vi "OSSP_Problem_Read.vi"(8 "error in (no error)":errorcluster, 11 "OSSP_Problem.lvclass In":refnum<class "OSSP_Problem.lvclass">) -> (0 "error out":errorcluster, 3 "OSSP_Problem.lvclass Out":refnum<class "OSSP_Problem.lvclass">)   [LabVIEW 2013, in "OSSP_Problem.lvclass"]
uses:
  OSSP_Problem.lvclass
  OSSP_Problem.lvclass/OSSP_Problem.ctl
panel:
  out "Array":u16[][](array[numeric])
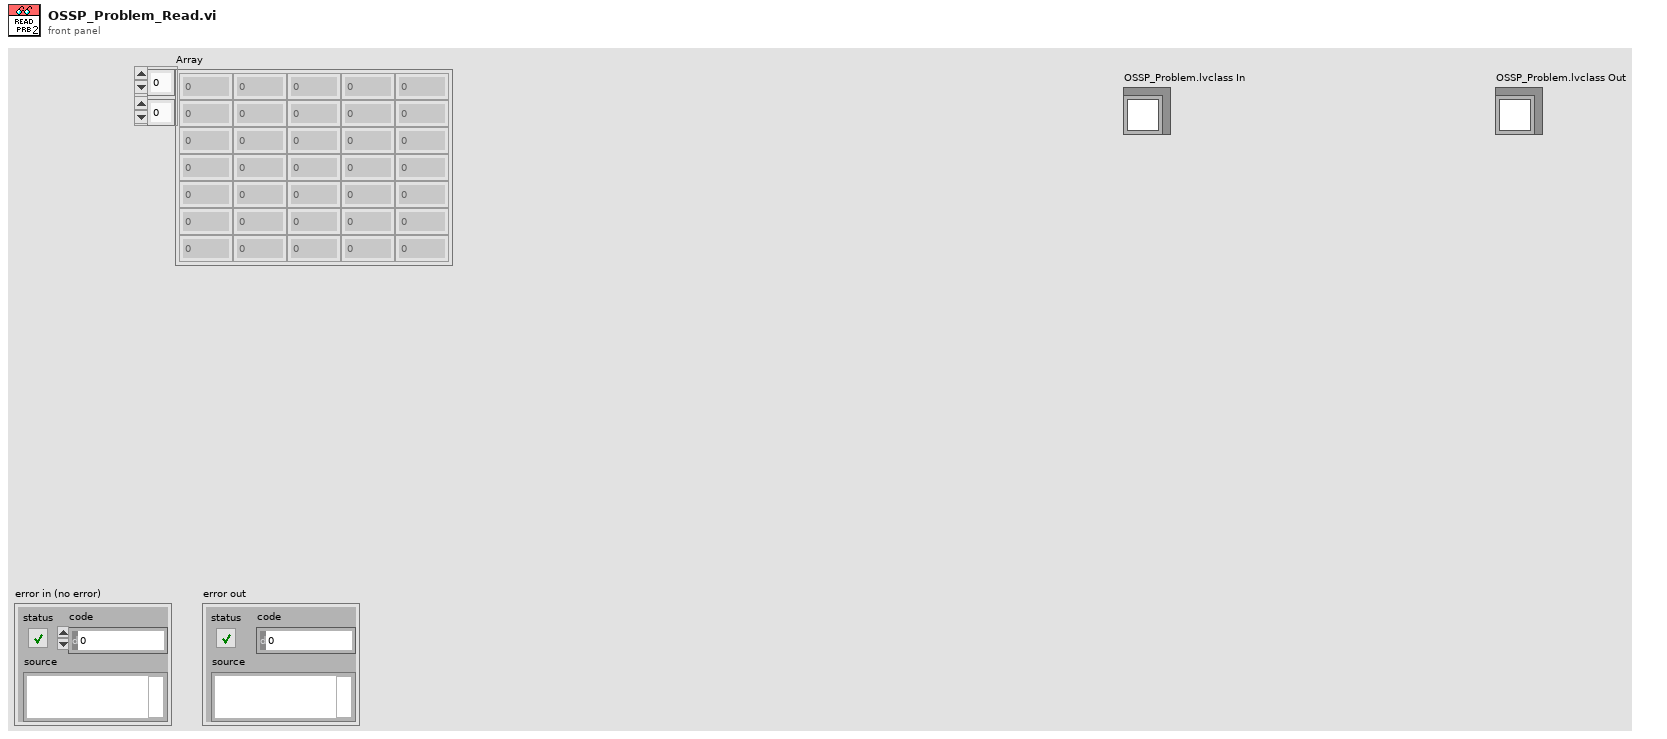
[diagram p1: front panel]
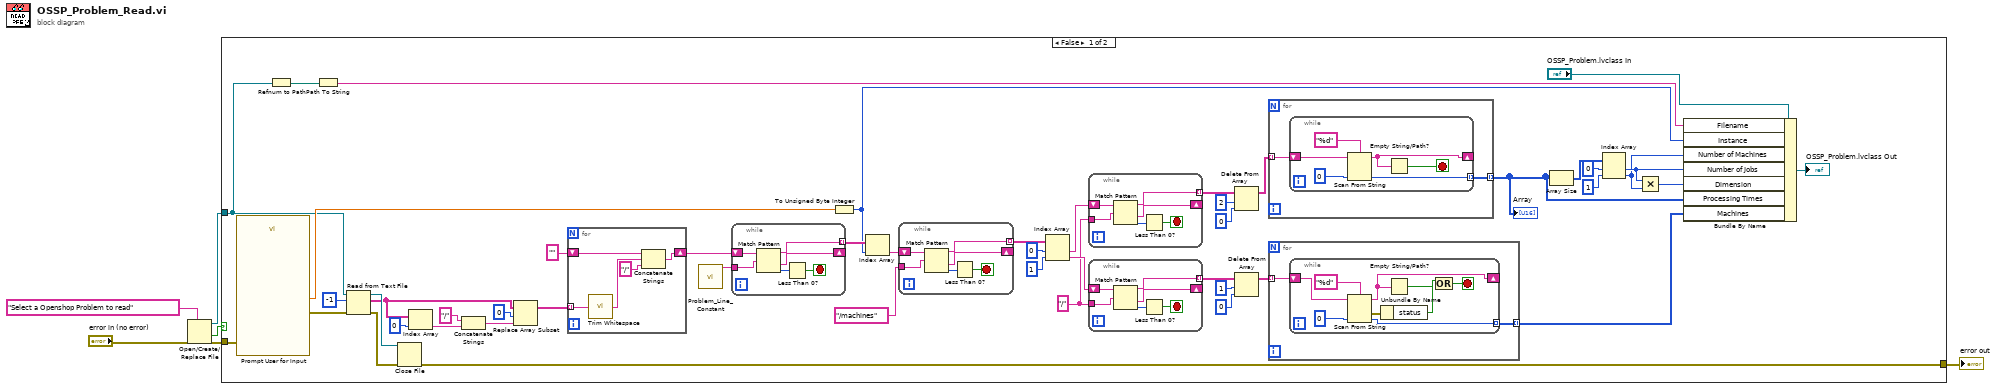
[diagram p0: block diagram]
diagram:
  n1 = Open/Create/Replace File(error in="error in (no error)", prompt="Select a Openshop Problem to read") -> (refnum out=w3:refnum<file>, cancelled=w2:bool, error out=w4:errorcluster)  [unwired: 4 in]
  n2 = case shown="False" w2 {
    tunnel: w4 -> [w51 w103]
    tunnel: w3 -> [w9 _]
    tunnel: [w10 w103] -> w1
    frame False {
      w27 = "/" ("Problem Line")
      n3 = call "Prompt User for Input"("error in (no error)"=w51) -> ("Instance Number"=w49:dbl, "error out"=w50:errorcluster)  [unwired: 16 in, 1 out]
      n4 = Refnum to Path(1:w9) -> (0:w8:path)
      n5 = Path To String(path=w8) -> (string=w7:string)
      n6 = Read from Text File(file (use dialog)=w9, count=-1, error in=w50) -> (refnum out=w53:refnum<file>, text=w44:string[], error out=w52:errorcluster)  [unwired: 1 in, 1 out]
      n7 = Close File(refnum=w53, error in=w52) -> (error out=w10:errorcluster)  [unwired: 1 out]
      n8 = Index Array(array=w44, index=0) -> (element=w47:string)
      n9 = Concatenate Strings("/" ("string"), w47) -> (w43:string)
      n10 = Replace Array Subset(array=w44, new element=w43, index=0) -> (w42:string[])
      n11 = for {
        tunnel: w42 -> [w94] mode=indexing
        shift-right: [w90] -> w40
        shift-left: "" -> [w93]
        n12 = call <vilib>:"Trim Whitespace.vi"("string"=w94) -> ("trimmed string"=w92:string)  [unwired: 1 in]
        n13 = Concatenate Strings(w93, w92, "/" ("string")) -> (w90:string)
      }
      n14 = call "Problem_Line_Constant.vi"() -> ("Problem Line"=w39:string)  [unwired: 11 in]
      n15 = while {
        tunnel: w39 -> [w88]
        shift-right: [w86] -> _
        shift-left: w40 -> [w89]
        tunnel: [w85] -> w38 mode=indexing
        stop <- w84 stop-if-true
        n16 = Match Pattern(string=w89, regular expression=w88) -> (before substring=w85:string, after substring=w86:string, offset past match=w87:i32)  [unwired: 1 in, 1 out]
        n17 = Less Than 0?(x=w87) -> (x < 0?=w84:bool)
      }
      n18 = To Unsigned Byte Integer(number=w49) -> (unsigned 8bit integer=w20:u8)
      n19 = Index Array(array=w38, index=w20) -> (element=w37:string)
      n20 = while {
        tunnel: "/machines" ("Problem Line") -> [w82]
        shift-right: [w80] -> _
        shift-left: w37 -> [w83]
        tunnel: [w79] -> w35 mode=indexing
        stop <- w78 stop-if-true
        n21 = Match Pattern(string=w83, regular expression=w82) -> (before substring=w79:string, after substring=w80:string, offset past match=w81:i32)  [unwired: 1 in, 1 out]
        n22 = Less Than 0?(x=w81) -> (x < 0?=w78:bool)
      }
      n23 = Index Array(array=w35, index #1=0 ("index"), index #2=1 ("index")) -> (element #1=w33:string, element #2=w28:string)
      n24 = while {
        tunnel: w27 -> [w76]
        shift-right: [w74] -> _
        shift-left: w33 -> [w77]
        tunnel: [w73] -> w32 mode=indexing
        stop <- w72 stop-if-true
        n25 = Match Pattern(string=w77, regular expression=w76) -> (before substring=w73:string, after substring=w74:string, offset past match=w75:i32)  [unwired: 1 in, 1 out]
        n26 = Less Than 0?(x=w75) -> (x < 0?=w72:bool)
      }
      n27 = while {
        tunnel: w27 -> [w70]
        shift-right: [w68] -> _
        shift-left: w28 -> [w71]
        tunnel: [w67] -> w26 mode=indexing
        stop <- w66 stop-if-true
        n28 = Match Pattern(string=w71, regular expression=w70) -> (before substring=w67:string, after substring=w68:string, offset past match=w69:i32)  [unwired: 1 in, 1 out]
        n29 = Less Than 0?(x=w69) -> (x < 0?=w66:bool)
      }
      n30 = Delete From Array(array=w32, length=2, index=0) -> (array with subset deleted=w23:string[])  [unwired: 1 out]
      n31 = Delete From Array(array=w26, length=1, index=0) -> (array with subset deleted=w22:string[])  [unwired: 1 out]
      n32 = for {
        tunnel: w23 -> [w96] mode=indexing
        tunnel: [w95] -> w12 mode=indexing
        n33 = while {
          shift-right: [w98] -> _
          shift-left: w96 -> [w102]
          tunnel: [w100] -> w95 mode=indexing
          stop <- w97 stop-if-true
          n34 = Scan From String(format string="%d", input string=w102, default 1=u16 0 ("default value 1")) -> (remaining string=w98:string, output 1=w100:u16)  [unwired: 2 in, 2 out]
          n35 = Empty String/Path?(string/path=w98) -> (empty?=w97:bool)
        }
      }
      "Array" <- w12
      n36 = for {
        tunnel: w22 -> [w56] mode=indexing
        tunnel: [w55] -> w11 mode=indexing
        n37 = while {
          shift-right: [w61] -> _
          shift-left: w56 -> [w65]
          tunnel: [w63] -> w55 mode=indexing
          stop <- w57 stop-if-true
          n38 = Scan From String(format string="%d", input string=w65, default 1=u16 0 ("default value 1")) -> (remaining string=w61:string, error out=w60:errorcluster, output 1=w63:u16)  [unwired: 2 in, 1 out]
          n39 = Unbundle By Name(w60) -> ("status"=w59:bool)
          n40 = Empty String/Path?(string/path=w61) -> (empty?=w58:bool)
          n41 = Or(x=w59, y=w58) -> (x .or. y?=w57:bool)
        }
      }
      n42 = Array Size(array=w12) -> (size(s)=w19:i32[])
      n43 = Index Array(array=w19, index #1=0 ("index"), index #2=1 ("index")) -> (element #1=w16:i32, element #2=w15:i32)
      n44 = Multiply(x=w16, y=w15) -> (x*y=w14:i32)
      n45 = Bundle By Name(cluster="OSSP_Problem.lvclass In", "Filename"=w7, "Instance"=w20, "Number of Machines"=w15, "Number of Jobs"=w16, "Dimension"=w14, "Processing Times"=w12, "Machines"=w11) -> (→"OSSP_Problem.lvclass Out":refnum<class "OSSP_Problem.lvclass">)
    }
    frame True {
    }
  }
  "error out" <- w1
